vi "Update Acquisition Hold-Off Points in Record.vi"(8 "Increment?":bool, 9 "Trigger Hold Off Ticks Finished":u16, 11 "Trigger Hold-Off Ticks":u16) -> (0 "Trigger Hold Off Ticks Finish":bool, 1 "Updated Trigger Hold Off Done":u16, 2 "Is Trigger Hold Off =0?":bool)   [LabVIEW 2014]
panel:
  # "Copyright 2014 Vidrio Technologies\nScanImage 5 software is licensed under the Apache License, Version 2.0 (the \"License\"); you may not use any files contained\nwithin the ScanImage 5 release except in compliance with the License. You may obtain a copy of the License at\n http://www.apache.org/licenses/LICENSE-2.0\nUnless required by applicable law or agreed to in writing, software distributed under the License is distributed on an\n\"AS IS\" BASIS, WITHOUT WARRANTIES OR CONDITIONS OF ANY KIND, either express or implied. See the License for the\n specific language governing permissions and limitations under the License."
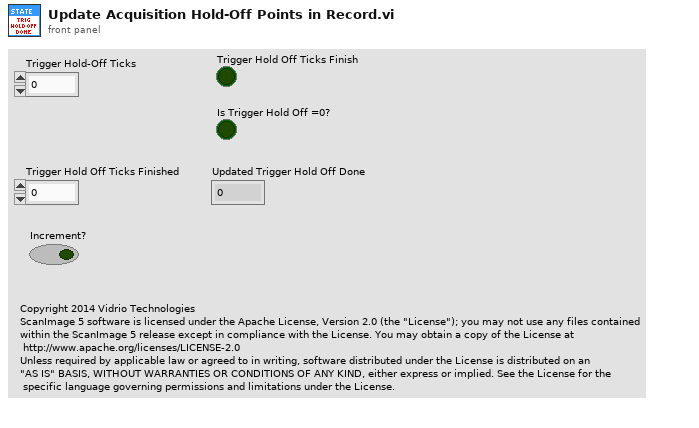
[diagram p1: front panel]
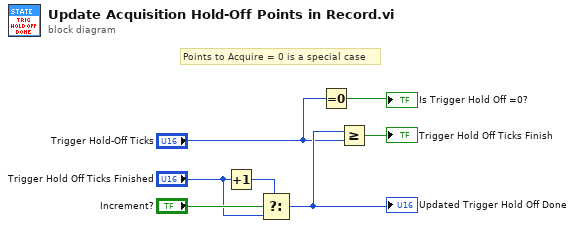
[diagram p0: block diagram]
diagram:
  # "Points to Acquire = 0 is a special case"
  n1 = Increment(x="Trigger Hold Off Ticks Finished") -> (x+1=w7:u16)
  n2 = Select(t=w7, s="Increment?", f="Trigger Hold Off Ticks Finished") -> (s? t:f=w4:u16)
  "Updated Trigger Hold Off Done" <- w4
  n3 = Equal To 0?(x="Trigger Hold-Off Ticks") -> (x = 0?=→"Is Trigger Hold Off =0?":bool)
  n4 = Greater Or Equal?(x=w4, y="Trigger Hold-Off Ticks") -> (x >= y?=→"Trigger Hold Off Ticks Finish":bool)
